vi "Member_Panel.vi"(8 "error in (no error)":errorcluster, 11 "MemberInfo in":refnum<class "MemberInfo.lvclass">) -> (0 "error out":errorcluster, 3 "MemberInfo out":refnum<class "MemberInfo.lvclass">)   [LabVIEW 2015, in "Member_Actor.lvlib"]
uses:
  Member_Actor.lvlib
  MemberInfo.lvclass
  Type Definitions/Main Ctl and VI ref.ctl
  MemberInfo.lvclass/MemberInfo.ctl
  <vilib>/Utility/error.llb/Error Cluster From Error Code.vi
  <vilib>/ErrorRing/Error Ring.xnode
panel:
  in  "Stop":bool
  in  "组别":enum16{"电控", "机械", "视觉"}(ring)
  in  "操作资料":bool caption="修改信息"
  in  "部门":string
  in  "点击上传照片":bool
  out "照片":picture
  in  "学号":string
  in  "学院":string
  in  "QQ":string
  in  "电话":string
  in  "邮箱":string
  in  "性别":enum16{"男", "女"}(ring)
  in  "年龄":dbl
  in  "姓名":string
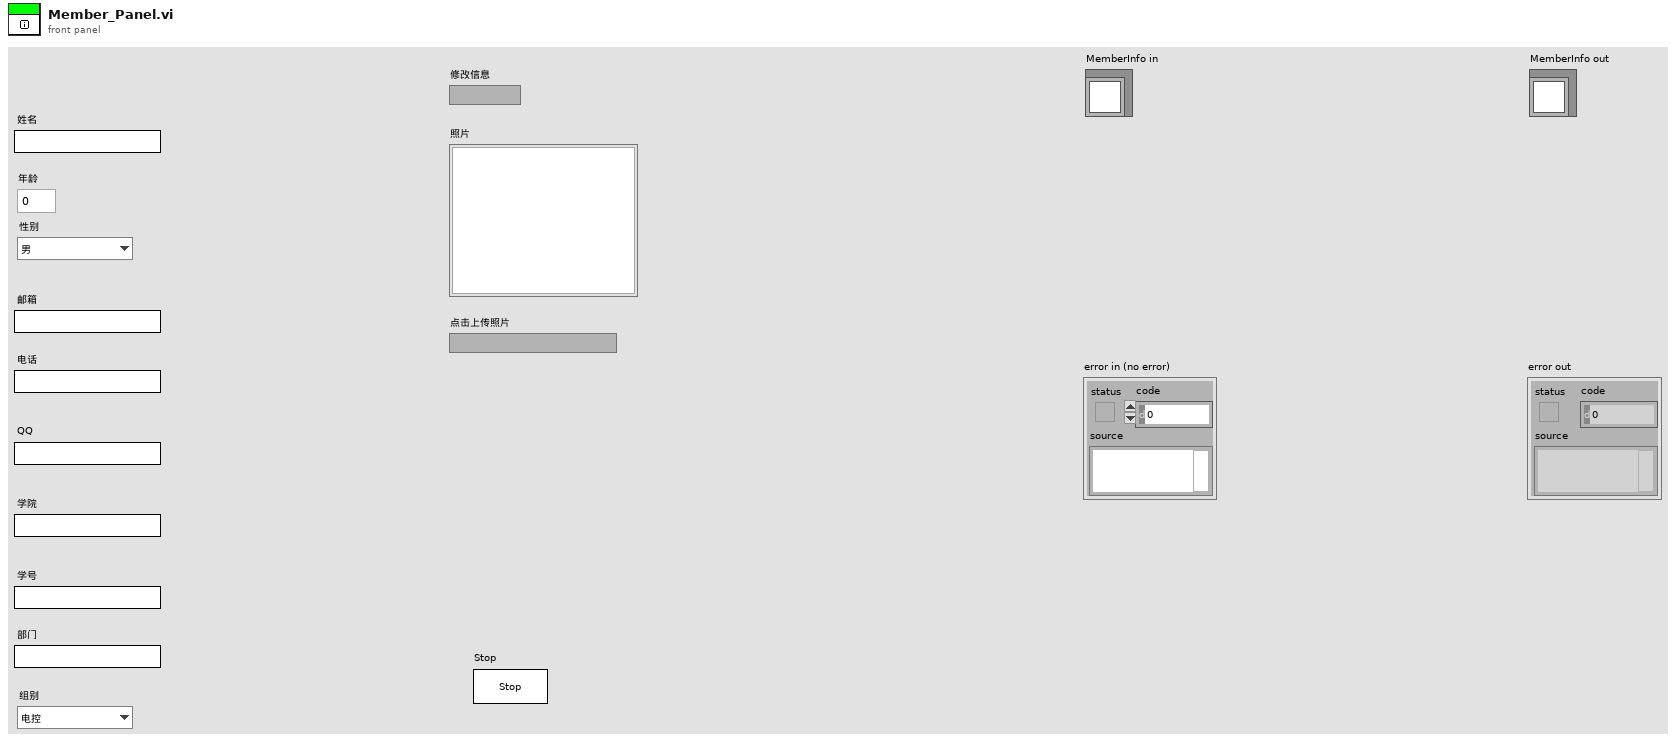
[diagram p1: front panel]
types:
  T1 = typedef "Member_Actor.lvlib/MemberInfo.lvclass/Main Ctl and VI ref.ctl" = cluster{"姓名":refnum<vi>, "年龄":refnum<vi>, "学号":refnum<vi>, "照片":refnum<vi>, "性别":refnum<vi>, "邮箱":refnum<vi>, "电话":refnum<vi>, "QQ":refnum<vi>, "学院":refnum<vi>, "点击上传照片":refnum<vi>, "操作资料":refnum<vi>, "部门":refnum<vi>, "组别":refnum<vi>}
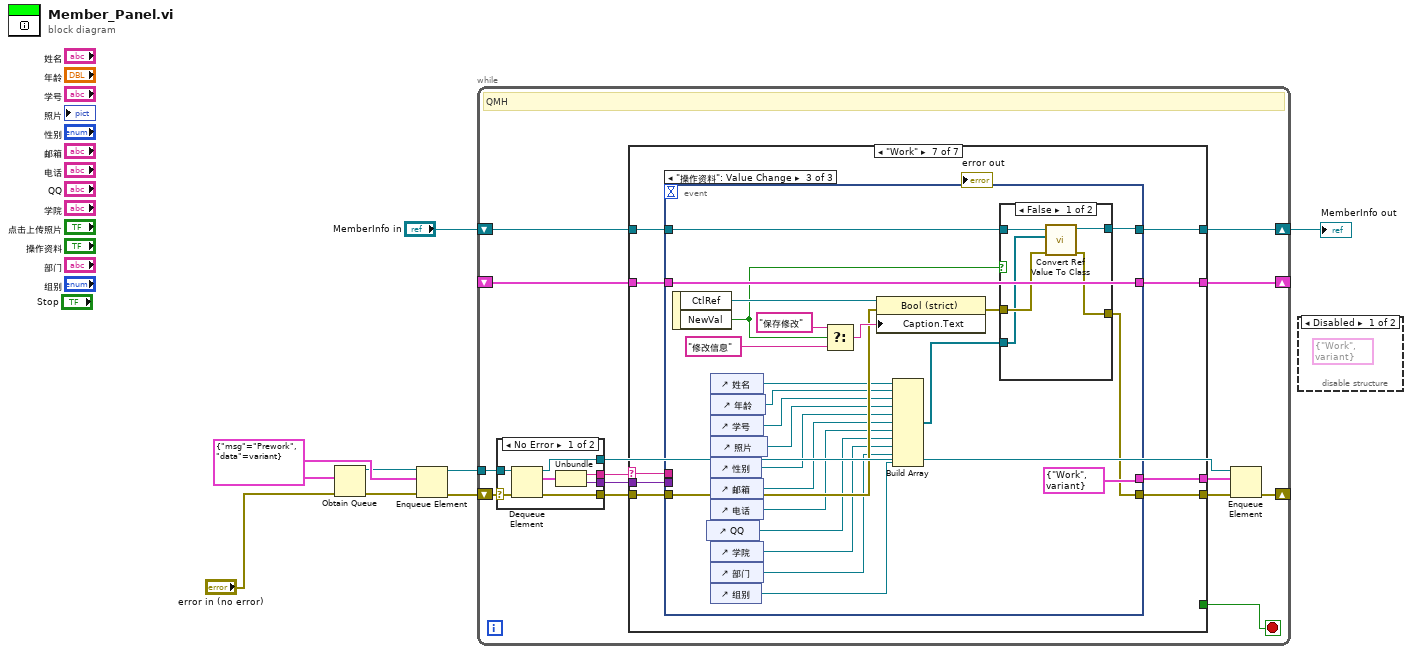
[diagram p0: block diagram]
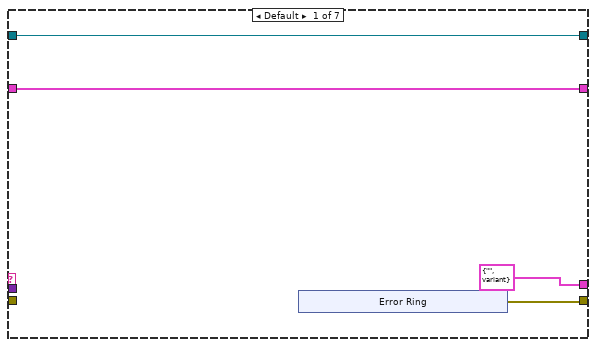
[diagram p3: hidden frame]
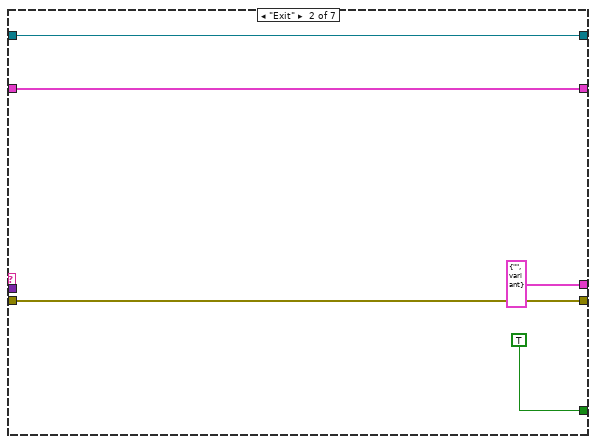
[diagram p4: hidden frame]
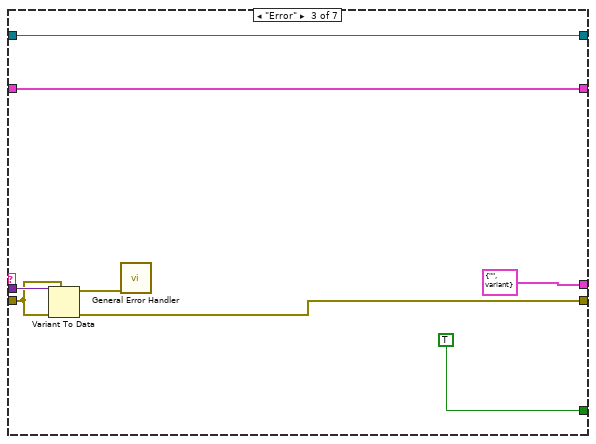
[diagram p5: hidden frame]
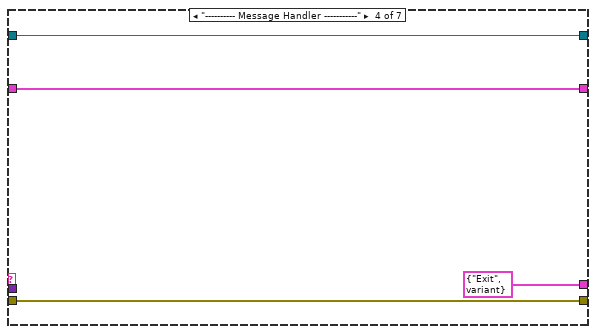
[diagram p6: hidden frame]
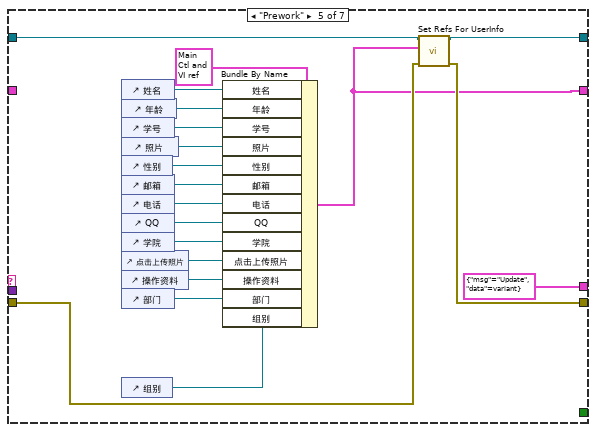
[diagram p7: hidden frame]
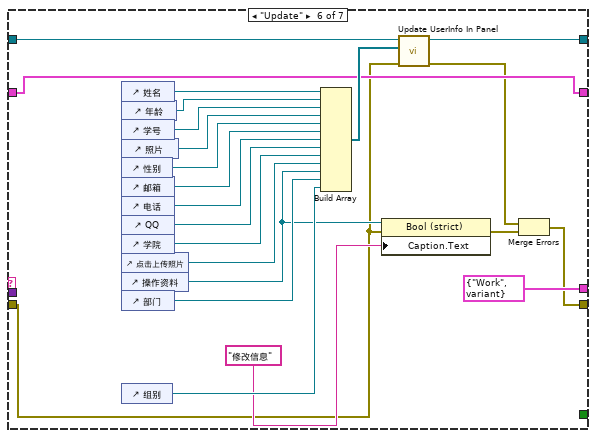
[diagram p8: hidden frame]
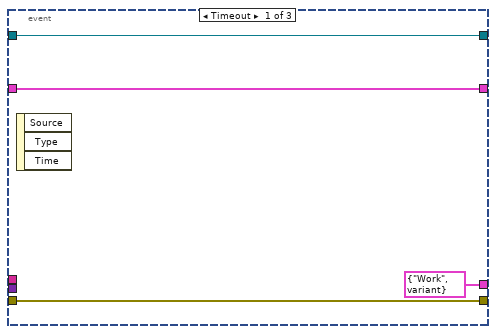
[diagram p9: hidden frame]
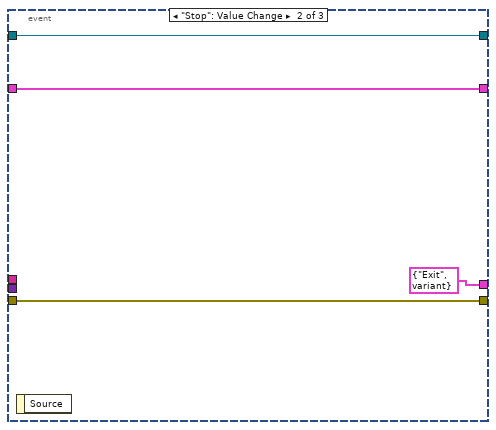
[diagram p10: hidden frame]
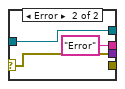
[diagram p12: hidden frame]
diagram:
  w6 = cluster{"msg":string, "data":variant} {"msg"="Prework", "data"=variant}
  n1 = Obtain Queue(element data type=w6, error in (no error)="error in (no error)") -> (queue out=w4:refnum<queue>, error out=w5:errorcluster)  [unwired: 3 in, 1 out]
  n2 = Enqueue Element(queue=w4, element=w6, error in (no error)=w5) -> (queue out=w7:refnum<queue>, error out=w8:errorcluster)  [unwired: 1 in, 1 out]
  n3 = while {
    tunnel: w7 -> [w21]
    shift-right: [w16] -> _
    shift-left: w8 -> [w22]
    shift-right: [w11] -> w1
    shift-left: "MemberInfo in" -> [w12]
    shift-right: [w10] -> _
    shift-left: _ -> [w9]
    stop <- w13 stop-if-true
    # "QMH"
    n4 = case shown="No Error" w22 {
      selector: w22 -> [w145 w149]
      tunnel: w21 -> [w146 w147]
      tunnel: [w144 _] -> w20
      tunnel: [w142 "Error" ("msg")] -> w19
      tunnel: [w141 w149] -> w18
      tunnel: [w140 w147] -> w15
      frame No Error {
        n5 = Dequeue Element(queue=w146, error in (no error)=w145) -> (queue out=w140:refnum<queue>, element=w143:cluster{"msg":string, "data":variant}, error out=w144:errorcluster)  [unwired: 1 in, 1 out]
        n6 = Unbundle(w143) -> ("msg"=w142:string, "data"=w141:variant)
      }
      frame Error {
      }
    }
    n7 = case shown="\"Work\"" w19 {
      selector: w19 -> [_ _ _ _ _ _ w98]
      tunnel: w20 -> [_ w36 w43 w48 w52 w72 w100]
      tunnel: w18 -> [_ _ w44 _ _ _ w99]
      tunnel: [w26 w36 w41 w48 w50 w69 w97] -> w17
      tunnel: [cluster{"msg":string, "data":variant} {"msg"="", "data"=variant} cluster{"msg":string, "data":variant} {"msg"="", "data"=variant} cluster{"msg":string, "data":variant} {"msg"="", "data"=variant} cluster{"msg":string, "data":variant} {"msg"="Exit", "data"=variant} cluster{"msg":string, "data":variant} {"msg"="Update", "data"=variant} cluster{"msg":string, "data":variant} {"msg"="Work", "data"=variant} w96] -> w14
      tunnel: [_ TRUE TRUE _ _ _ _] -> w13
      tunnel: w12 -> [w24 w33 w38 w46 w53 w78 w95]
      tunnel: [w24 w33 w38 w46 w51 w76 w94] -> w11
      tunnel: [w23 w32 w37 w45 w49 w75 w92] -> w10
      tunnel: w9 -> [w23 w32 w37 w45 _ w75 w93]
      frame Default {
        n8 = xnode "Error Ring"() -> ("error out"=w26:errorcluster)
      }
      frame "Exit" {
      }
      frame "Error" {
        n9 = Variant To Data(error in=w43, type=w43, Variant=w44) -> (data=w42:errorcluster, error out=w41:errorcluster)
        n10 = call <vilib>:"General Error Handler.vi"("error in (no error)"=w42) -> ()  [unwired: 10 in, 5 out]
      }
      frame "---------- Message Handler -----------" {
      }
      frame "Prework" {
        n11 = control-ref of="姓名"() -> (w66:refnum<vi>)
        n12 = control-ref of="年龄"() -> (w65:refnum<vi>)
        n13 = control-ref of="学号"() -> (w64:refnum<vi>)
        n14 = control-ref of="照片"() -> (w63:refnum<vi>)
        n15 = control-ref of="性别"() -> (w62:refnum<vi>)
        n16 = control-ref of="邮箱"() -> (w61:refnum<vi>)
        n17 = control-ref of="电话"() -> (w60:refnum<vi>)
        n18 = control-ref of="QQ"() -> (w59:refnum<vi>)
        n19 = control-ref of="学院"() -> (w58:refnum<vi>)
        n20 = control-ref of="点击上传照片"() -> (w57:refnum<vi>)
        n21 = control-ref of="操作资料"() -> (w56:refnum<vi>)
        n22 = control-ref of="部门"() -> (w55:refnum<vi>)
        n23 = control-ref of="组别"() -> (w54:refnum<vi>)
        n24 = Bundle By Name(cluster=T1 {"姓名"=refnum, "年龄"=refnum, "学号"=refnum, "照片"=refnum, "性别"=refnum, "邮箱"=refnum, "电话"=refnum, "QQ"=refnum, "学院"=refnum, "点击上传照片"=refnum, "操作资料"=refnum, "部门"=refnum, "组别"=refnum} ("Refs"), "姓名"=w66, "年龄"=w65, "学号"=w64, "照片"=w63, "性别"=w62, "邮箱"=w61, "电话"=w60, "QQ"=w59, "学院"=w58, "点击上传照片"=w57, "操作资料"=w56, "部门"=w55, "组别"=w54) -> (w49:T1)
        n25 = call "Set Refs For UserInfo.vi"("error in (no error)"=w52, "Refs"=w49, "MemberInfo in"=w53) -> ("error out"=w50:errorcluster, "MemberInfo out"=w51:refnum<class "MemberInfo.lvclass">)  [unwired: 7 in]
      }
      frame "Update" {
        n26 = control-ref of="姓名"() -> (w81:refnum<vi>)
        n27 = control-ref of="年龄"() -> (w82:refnum<vi>)
        n28 = control-ref of="学号"() -> (w83:refnum<vi>)
        n29 = control-ref of="照片"() -> (w84:refnum<vi>)
        n30 = control-ref of="性别"() -> (w85:refnum<vi>)
        n31 = control-ref of="邮箱"() -> (w86:refnum<vi>)
        n32 = control-ref of="电话"() -> (w87:refnum<vi>)
        n33 = control-ref of="QQ"() -> (w88:refnum<vi>)
        n34 = control-ref of="学院"() -> (w89:refnum<vi>)
        n35 = control-ref of="点击上传照片"() -> (w90:refnum<vi>)
        n36 = control-ref of="操作资料"() -> (w74:refnum<vi>)
        n37 = control-ref of="部门"() -> (w80:refnum<vi>)
        n38 = control-ref of="组别"() -> (w79:refnum<vi>)
        n39 = Build Array(w81, w82, w83, w84, w85, w86, w87, w88, w89, w90, w74, w80, w79) -> (w77:refnum<vi>[])
        n40 = property class="Bool (strict)"(reference=w74, error in=w72, "Caption.Text"="修改信息") -> (error out=w71:errorcluster)  [unwired: 1 out]
        n41 = call "Update UserInfo In Panel.vi"("error in (no error)"=w72, "UI Ref"=w77, "MemberInfo in"=w78) -> ("error out"=w70:errorcluster, "MemberInfo out"=w76:refnum<class "MemberInfo.lvclass">)  [unwired: 6 in, 1 out]
        n42 = Merge Errors(w70, w71) -> (w69:errorcluster)
      }
      frame "Work" {
        n43 = event shown="[2] \"操作资料\": Value Change" {
          selector: _ -> [_ _ _]
          dyn-events: _ -> [_ _ _]
          timeout: _ -> [_ _ _]
          tunnel: w100 -> [w104 w108 w127]
          tunnel: w99 -> [_ _ _]
          tunnel: w98 -> [_ _ _]
          tunnel: [w104 w108 w110] -> w97
          tunnel: [cluster{"msg":string, "data":variant} {"msg"="Work", "data"=variant} cluster{"msg":string, "data":variant} {"msg"="Exit", "data"=variant} cluster{"msg":string, "data":variant} {"msg"="Work", "data"=variant}] -> w96
          tunnel: w95 -> [w102 w106 w124]
          tunnel: [w102 w106 w109] -> w94
          tunnel: w93 -> [w101 w105 w132]
          tunnel: [w101 w105 w132] -> w92
          event Timeout {
            n44 = event-data() -> ()  [unwired: 1 in, 3 out]
          }
          event "Stop": Value Change {
            n45 = event-data() -> ()  [unwired: 1 in, 1 out]
          }
          event "操作资料": Value Change {
            n46 = event-data() -> ("CtlRef"=w129:refnum<vi>, "NewVal"=w125:bool)  [unwired: 1 in]
            n47 = control-ref of="QQ"() -> (w116:refnum<vi>)
            n48 = control-ref of="姓名"() -> (w123:refnum<vi>)
            n49 = control-ref of="年龄"() -> (w122:refnum<vi>)
            n50 = control-ref of="学号"() -> (w121:refnum<vi>)
            n51 = control-ref of="照片"() -> (w120:refnum<vi>)
            n52 = control-ref of="性别"() -> (w119:refnum<vi>)
            n53 = control-ref of="邮箱"() -> (w118:refnum<vi>)
            n54 = control-ref of="电话"() -> (w117:refnum<vi>)
            n55 = control-ref of="学院"() -> (w115:refnum<vi>)
            n56 = control-ref of="部门"() -> (w114:refnum<vi>)
            n57 = control-ref of="组别"() -> (w113:refnum<vi>)
            n58 = Select(t="保存修改", s=w125, f="修改信息") -> (s? t:f=w128:string)
            n59 = property class="Bool (strict)"(reference=w129, error in=w127, "Caption.Text"=w128) -> (error out=w111:errorcluster)  [unwired: 1 out]
            n60 = Build Array(w123, w122, w121, w120, w119, w118, w117, w116, w115, w114, w113) -> (w112:refnum<vi>[])
            n61 = case shown="False" w125 {
              tunnel: w124 -> [w137 w139]
              tunnel: w112 -> [w135 _]
              tunnel: w111 -> [w136 w138]
              tunnel: [w134 w138] -> w110
              tunnel: [w133 w139] -> w109
              frame False {
                n62 = call "Convert Ref Value To Class.vi"("error in (no error)"=w136, "Main Ctls and VI Refs"=w135, "MemberInfo in"=w137) -> ("error out"=w134:errorcluster, "MemberInfo out"=w133:refnum<class "MemberInfo.lvclass">)  [unwired: 7 in]
              }
              frame True {
              }
            }
          }
        }
      }
    }
    n63 = Enqueue Element(queue=w15, element=w14, error in (no error)=w17) -> (error out=w16:errorcluster)  [unwired: 1 in, 2 out]
  }
  "MemberInfo out" <- w1
  n64 = disable-structure shown="Disabled" {
    frame Disabled {
      (unwired) cluster{"msg":string, "data":variant} {"msg"="Work", "data"=variant}
    }
    frame Enabled {
    }
  }
